vi "GenerateSineProfile.vi"(4 "Fixed Source Delay of":dbl, 6 "Amplitude":dbl, 7 "DC offset":dbl, 9 "Frequency":dbl, 10 "Samples per Sine":u16, 11 "Amount of Itterations":i32) -> (1 "Time to Plot":dbl[](array[numeric]), 2 "Apperature Time":dbl, 3 "Voltage":dbl[](array[numeric]))   [LabVIEW 2023]
panel:
  out "Sine Ref":dbl[](graph)
  out "Stimulus Profile":cluster{"X":dbl, "Y":dbl}[](graph)
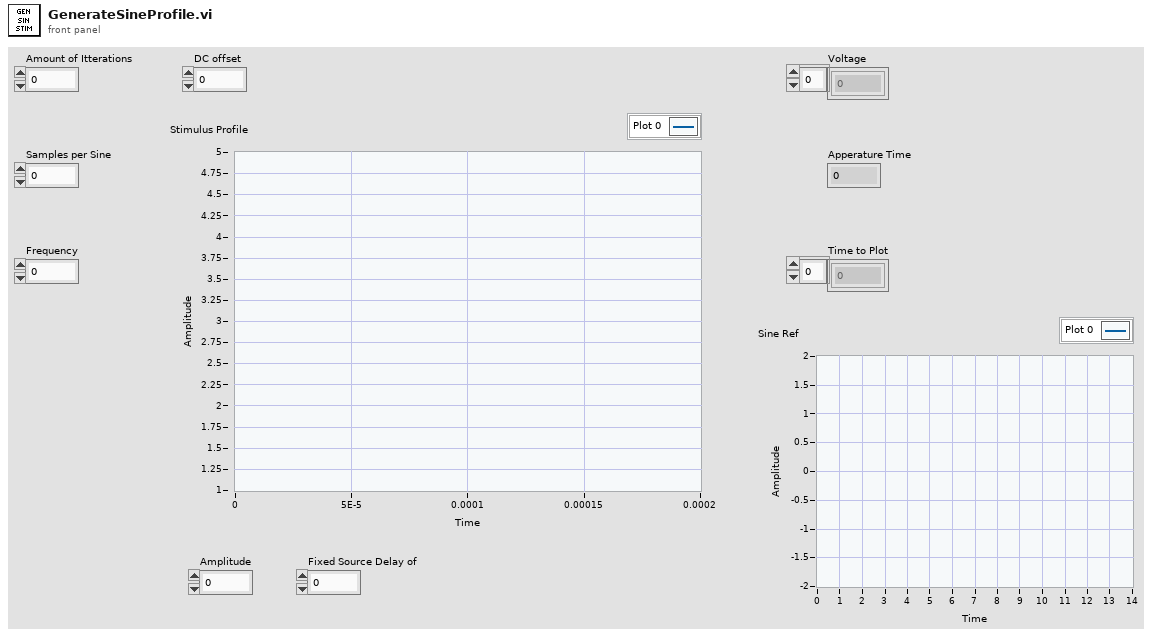
[diagram p1: front panel]
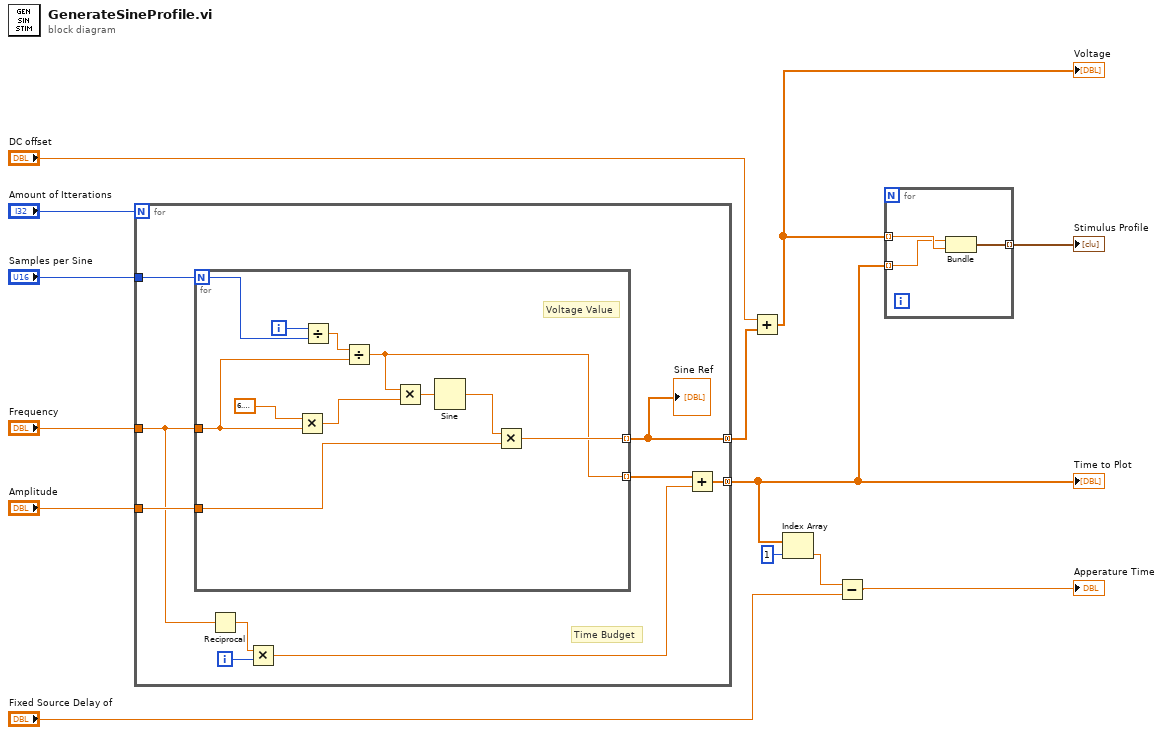
[diagram p0: block diagram]
diagram:
  n1 = for {
    N: "Amount of Itterations" -> [_]
    tunnel: "Samples per Sine" -> [w22]
    tunnel: "Amplitude" -> [w21]
    tunnel: [w14] -> w4 mode=concatenating
    tunnel: "Frequency" -> [w16]
    tunnel: [w17] -> w3 mode=concatenating
    i -> [w20]
    # "Time Budget"
    n2 = for {
      N: w22 -> [w28]
      tunnel: w21 -> [w33]
      tunnel: [w32] -> w14 mode=indexing
      tunnel: w16 -> [w24]
      tunnel: [w23] -> w18 mode=indexing
      i -> [w26]
      # "Voltage Value"
      n3 = Multiply(x=6.283185307179586, y=w24) -> (x*y=w30:dbl)
      n4 = Divide(x=w26, y=w28) -> (x/y=w25:dbl)
      n5 = Divide(x=w25, y=w24) -> (x/y=w23:dbl)
      n6 = Multiply(x=w23, y=w30) -> (x*y=w29:dbl)
      n7 = Sine(x=w29) -> (sin(x)=w31:dbl)
      n8 = Multiply(x=w31, y=w33) -> (x*y=w32:dbl)
    }
    "Sine Ref" <- w14
    n9 = Reciprocal(x=w16) -> (1/x=w15:dbl)
    n10 = Multiply(x=w15, y=w20) -> (x*y=w19:dbl)
    n11 = Add(x=w18, y=w19) -> (x+y=w17:dbl[])
  }
  "Time to Plot" <- w3
  n12 = Add(x="DC offset", y=w4) -> (x+y=w6:dbl[])
  "Voltage" <- w6
  n13 = Index Array(array=w3, index=1) -> (element=w1:dbl)
  n14 = Subtract(x=w1, y="Fixed Source Delay of") -> (x-y=→"Apperature Time":dbl)
  n15 = for {
    tunnel: w6 -> [w36] mode=indexing
    tunnel: w3 -> [w35] mode=indexing
    tunnel: [w34] -> w5 mode=indexing
    n16 = Bundle(w35, w36) -> (w34:cluster{dbl, dbl})  [unwired: 1 in]
  }
  "Stimulus Profile" <- w5
